vi "ViewData.vi"() -> ()   [LabVIEW 2024]
uses:
  <vilib>/drjdpowell/SQLite Library/SQL Connection/Open (path).vi
  <vilib>/drjdpowell/SQLite Library/SQL Connection/Open (string).vi
  <vilib>/AdvancedString/Path To Command Line String.vi
  <vilib>/drjdpowell/SQLite Library/SQL Connection/Execute SQL (1D String).vi
  <vilib>/drjdpowell/SQLite Library/SQL Connection/Execute SQL (DBL results).vi
  <vilib>/Utility/file.llb/Write Delimited Spreadsheet (DBL).vi
  <vilib>/drjdpowell/SQLite Library/SQL Connection/Connection.lvclass
  <vilib>/drjdpowell/SQLite Library/SQLite.lvlib
panel:
  out "length":i32
  in  "Export Excel":bool
  in  "Export Image Pressure":bool
  in  "Export Excel Pressure":bool
  in  "Export Image Fan":bool
  in  "Export Excel Fan":bool
  out "Data":dbl[][](array[numeric])
  out "Pressure":cluster{dbl[], "Data Table":dbl[]}[](graph)
  out "Fan":cluster{dbl[], "Result Set":dbl[]}[](graph)
  in  "Time":i32(listbox)
  in  "Date":string(combo)
  in  "stop":bool
  out "Time2DArray":string[][](array[string])
  out "DateArray":string[](array[string])
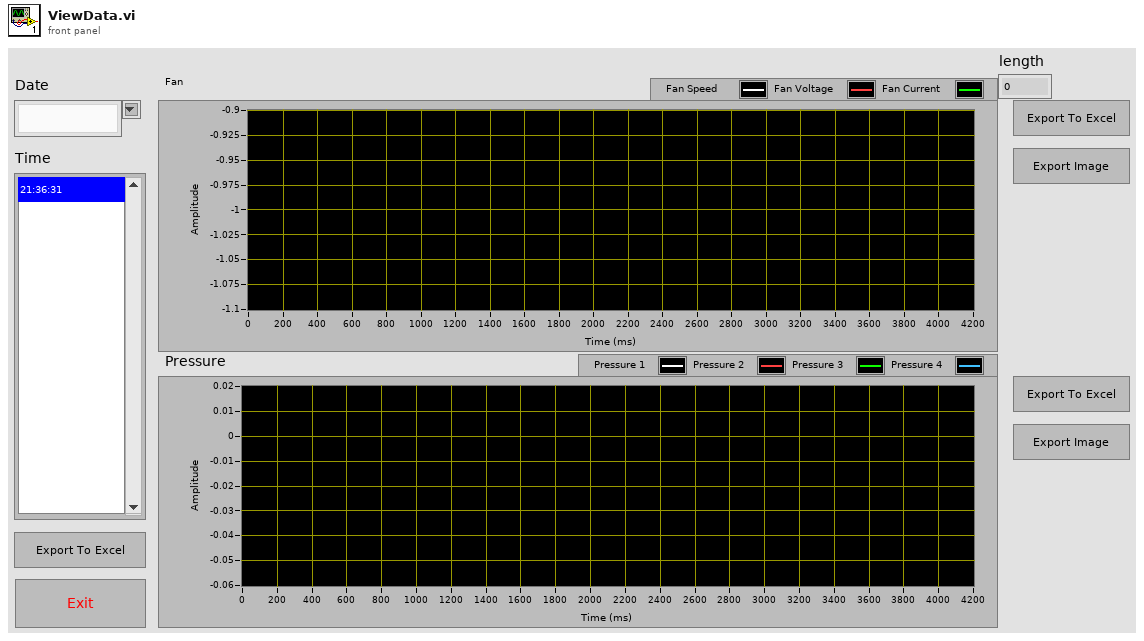
[diagram p1: front panel]
types:
  T1 = enum16{"New or existing", "Existing", "Read only"}
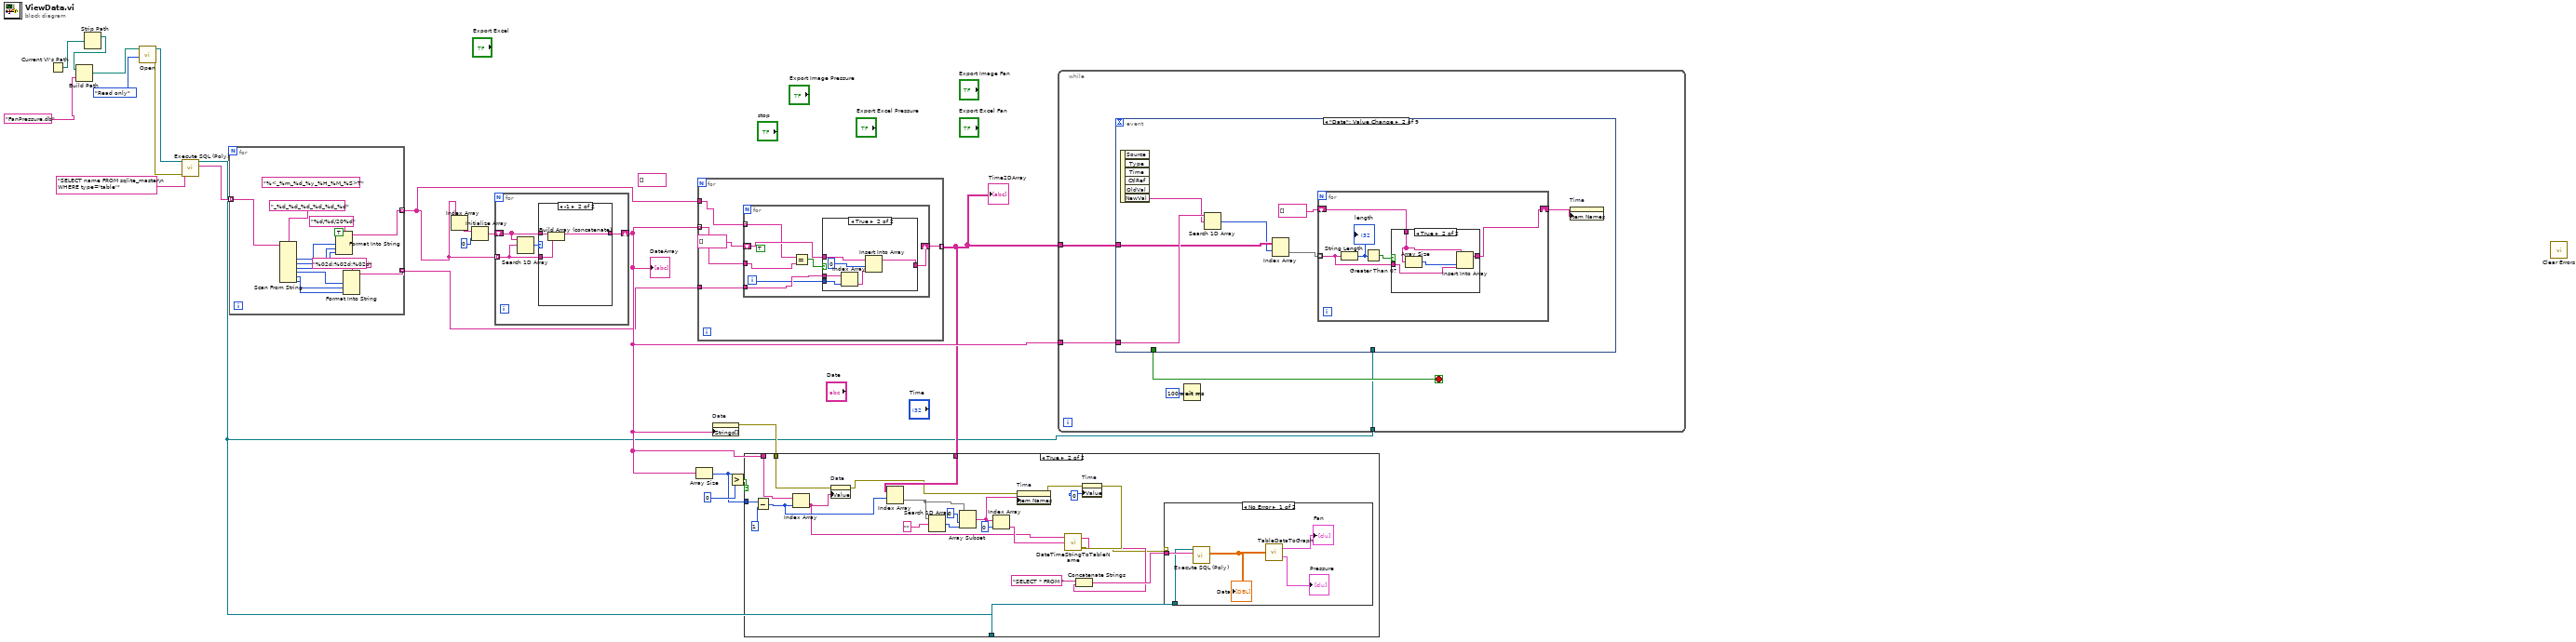
[diagram p0: block diagram]
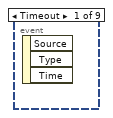
[diagram p4: hidden frame]
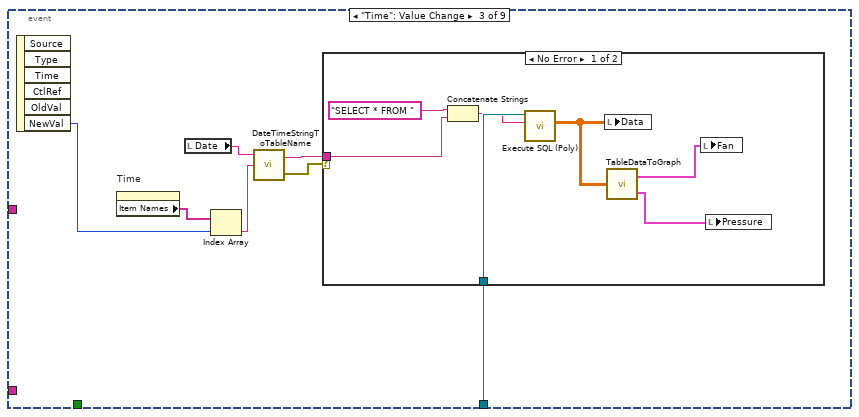
[diagram p6: hidden frame]
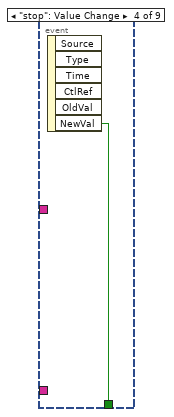
[diagram p8: hidden frame]
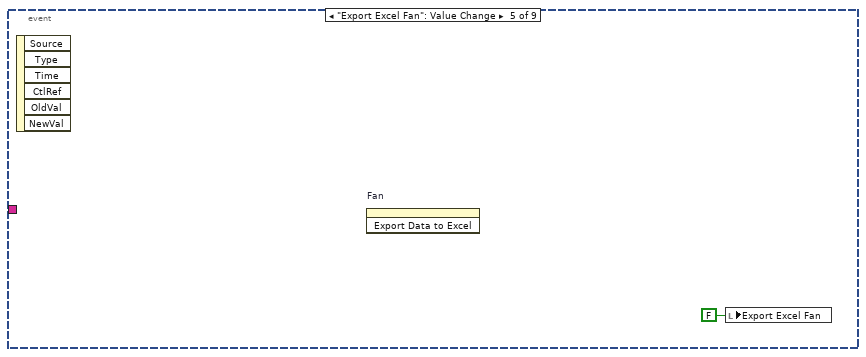
[diagram p9: hidden frame]
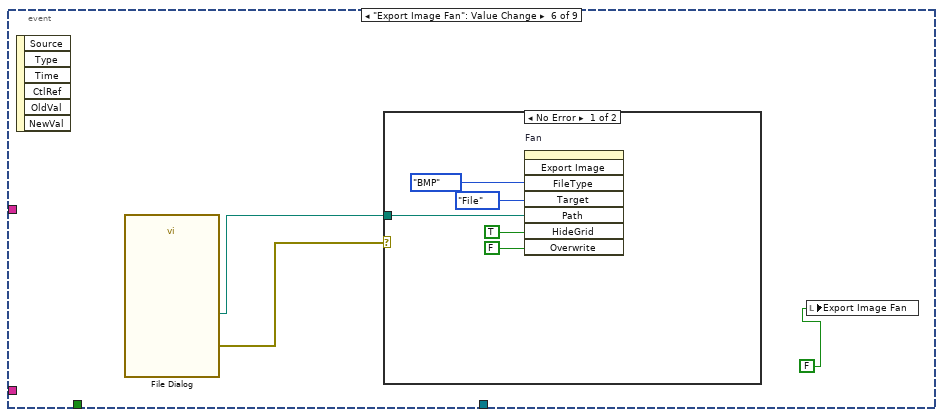
[diagram p10: hidden frame]
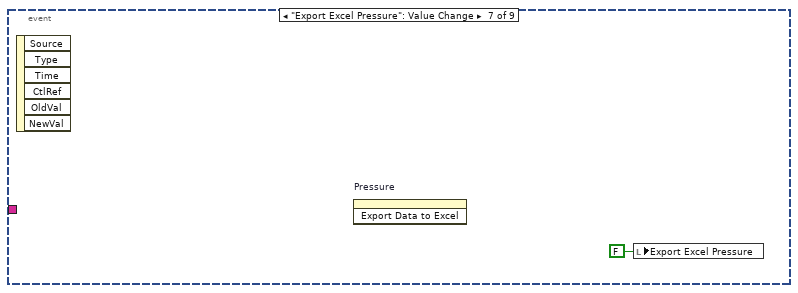
[diagram p12: hidden frame]
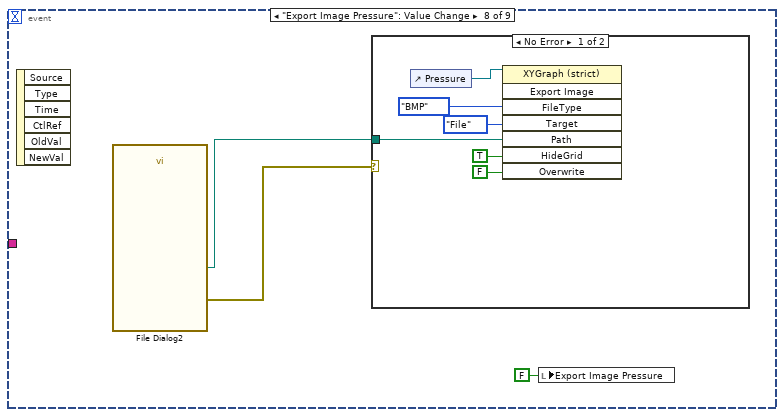
[diagram p13: hidden frame]
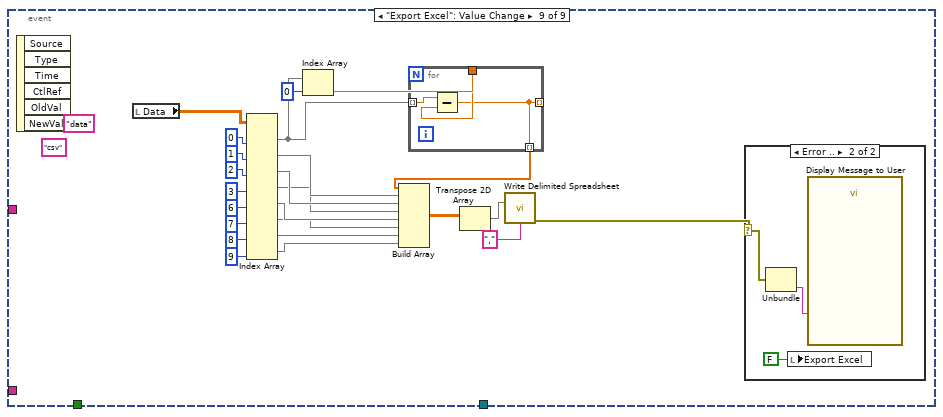
[diagram p15: hidden frame]
diagram:
  (unwired) string[] [] ("Child Text")
  n1 = Current VI's Path() -> (path=w19:path)
  n2 = Strip Path(path=w19) -> (stripped path=w17:path)  [unwired: 1 out]
  n3 = Build Path(base path=w17, name or relative path="FanPressure.db" ("db file")) -> (appended path=w16:path)
  n4 = call-poly <vilib>:"Open.vi"("File Option"=T1."Read only", "db file"=w16) -> ("error out"=w14:errorcluster, "SQLite Connection"=w15:refnum<class "Connection.lvclass">)  [unwired: 8 in]
  n5 = call-poly <vilib>:"Execute SQL (Poly).vi"("error in (no error)"=w14, "SQL"="SELECT name FROM sqlite_master\n    WHERE type='table'", "SQLite Connection in"=w15) -> ("Result Set"=w10:string[], "SQLite Connection"=w1:refnum<class "Connection.lvclass">)  [unwired: 5 in, 2 out]
  n6 = for {
    tunnel: w10 -> [w33] mode=indexing
    tunnel: [w27] -> w3 mode=indexing
    tunnel: [w22] -> w2 mode=indexing
    (unwired) TRUE ("want seconds? (F)")
    (unwired) "%<_%m_%d_%y_%H_%M_%S>T" ("format string")
    n7 = Scan From String(format string="_%d_%d_%d_%d_%d_%d", input string=w33) -> (output 1=w30:i32, output 2=w29:i32, output 3=w28:i32, output 4=w26:i32, output 5=w25:i32, output 6=w24:i32)  [unwired: 8 in, 3 out]
    n8 = Format Into String(format string="%d/%d/20%d", w30, w29, w28) -> (resulting string=w27:string)  [unwired: 2 in, 1 out]
    n9 = Format Into String(format string="%02d:%02d:%02d", w26, w25, w24) -> (resulting string=w22:string)  [unwired: 2 in, 1 out]
  }
  n10 = Index Array(array=w3) -> (element=w11:string)  [unwired: 1 in]
  n11 = Initialize Array(w11, 0 ("Dimension Size")) -> (w12:string[])
  n12 = for {
    tunnel: w3 -> [w36] mode=indexing
    shift-right: [w34] -> w6
    shift-left: w12 -> [w35]
    n13 = Search 1D Array(1D array=w35, element=w36) -> (index of element=w37:i32)  [unwired: 1 in]
    n14 = case shown="-1" w37 {
      tunnel: w36 -> [_ w41]
      tunnel: [w38 w39] -> w34
      tunnel: w35 -> [w38 w40]
      frame Default {
      }
      frame -1 {
        n15 = Build Array (concatenate)(w40, w41) -> (w39:string[])
      }
    }
  }
  "DateArray" <- w6
  n16 = Array Size(array=w6) -> (size(s)=w5:i32)
  n17 = for {
    tunnel: w6 -> [w46] mode=indexing
    tunnel: [w44] -> w4 mode=indexing
    tunnel: w3 -> [w43]
    tunnel: w2 -> [w42]
    n18 = for {
      tunnel: w46 -> [w53]
      shift-right: [w51] -> w44
      shift-left: string[] [] ("Child Text") -> [w52]
      tunnel: w43 -> [w49] mode=indexing
      tunnel: w42 -> [w48]
      i -> [w47]
      (unwired) TRUE ("want seconds? (F)")
      n19 = Equal?(x=w49, y=w53) -> (x = y?=w50:bool)
      n20 = case shown="True" w50 {
        tunnel: w52 -> [w54 w59]
        tunnel: [w54 w58] -> w51
        tunnel: w48 -> [_ w56]
        tunnel: w47 -> [_ w57]
        frame False {
        }
        frame True {
          n21 = Index Array(array=w56, index=w57) -> (element=w55:string)
          n22 = Insert Into Array(array=w59, index=0, new element=w55) -> (w58:string[])
        }
      }
    }
  }
  "Time2DArray" <- w4
  n23 = property on="Date" class="CmbBox"("Strings[]"=w6) -> (error out=w7:errorcluster)  [unwired: 2 in, 1 out]
  n24 = Greater?(x=w5, y=0) -> (0:w8:bool)
  n25 = case shown="True" w8 {
    tunnel: w7 -> [_ w82]
    tunnel: w6 -> [_ w79]
    tunnel: w5 -> [_ w81]
    tunnel: w4 -> [_ w78]
    tunnel: w1 -> [_ w71]
    frame False {
    }
    frame True {
      n26 = Subtract(x=w81, y=1) -> (x-y=w77:i32)
      n27 = Index Array(array=w79, index=w77) -> (element=w69:string)
      n28 = property on="Date" class="CmbBox"(error in=w82, "Value"=w69) -> (error out=w76:errorcluster)  [unwired: 1 in, 1 out]
      n29 = Index Array(array=w78, index (row)=w77) -> (element=w64:string[])  [unwired: 1 in]
      n30 = Search 1D Array(1D array=w64, element="") -> (index of element=w62:i32)  [unwired: 1 in]
      n31 = Array Subset(array=w64, index=0, length=w62) -> (w61:string[])
      n32 = Index Array(array=w61, index=0) -> (element=w70:string)
      n33 = property on="Time" class="LstBox (strict)"(error in=w76, "Item Names"=w61) -> (error out=w68:errorcluster)  [unwired: 1 in, 1 out]
      n34 = call "DateTimeStringToTableName.vi"("error in"=w68, "Time String"=w70, "Date String"=w69) -> ("error out"=w66:errorcluster, "Table Name"=w67:string)
      n35 = Concatenate Strings("SELECT * FROM " ("SQL"), w67) -> (w72:string)
      n36 = property on="Time" class="LstBox (strict)"(error in=w68, "Value"=0 ("Time")) -> ()  [unwired: 1 in, 2 out]
      n37 = case shown="No Error" w66 {
        tunnel: w72 -> [w87 _]
        tunnel: w71 -> [w83 _]
        frame No Error {
          n38 = call-poly <vilib>:"Execute SQL (Poly).vi"("SQL"=w87, "SQLite Connection in"=w83) -> ("Result Set"=w84:dbl[][])  [unwired: 6 in, 3 out]
          "Data" <- w84
          n39 = call "TableDataToGraph.vi"("Data Table"=w84) -> ("Speed Graph"=→"Fan":cluster{dbl[], "Data Table":dbl[]}[], "Pressure Graph"=→"Pressure":cluster{dbl[], "Data Table":dbl[]}[])
        }
        frame Error {
        }
      }
    }
  }
  n40 = while {
    tunnel: w6 -> [w91]
    tunnel: w4 -> [w90]
    tunnel: w1 -> [w88]
    stop <- w89 stop-if-true
    n41 = event shown="[1] \"Date\": Value Change" {
      selector: _ -> [_ _ _ _ _ _ _ _ _]
      dyn-events: _ -> [_ _ _ _ _ _ _ _ _]
      timeout: _ -> [_ _ _ _ _ _ _ _ _]
      tunnel: w91 -> [_ w99 _ _ _ _ _ _ _]
      tunnel: w90 -> [_ w97 _ _ _ _ _ _ _]
      tunnel: [_ _ _ w124 _ _ _ _ _] -> w89
      tunnel: w88 -> [_ _ w114 _ _ _ _ _ _]
      event Timeout {
        n42 = event-data() -> ()  [unwired: 1 in, 3 out]
      }
      event "Date": Value Change {
        n43 = event-data() -> ("NewVal"=w98:string)  [unwired: 1 in, 5 out]
        n44 = Search 1D Array(1D array=w99, element=w98) -> (index of element=w96:i32)  [unwired: 1 in]
        n45 = Index Array(array=w97, index (row)=w96) -> (element=w95:string[])  [unwired: 1 in]
        n46 = for {
          tunnel: w95 -> [w101] mode=indexing
          shift-right: [w100] -> w93
          shift-left: string[] [] ("Item Names") -> [w102]
          n47 = String Length(string=w101) -> (length=w104:i32)
          "length" <- w104
          n48 = Greater Than 0?(x=w104) -> (x > 0?=w103:bool)
          n49 = case shown="True" w103 {
            tunnel: w102 -> [w105 w108]
            tunnel: w101 -> [_ w109]
            tunnel: [w105 w107] -> w100
            frame False {
            }
            frame True {
              n50 = Array Size(array=w108) -> (size(s)=w106:i32)
              n51 = Insert Into Array(array=w108, index=w106, new element=w109) -> (w107:string[])
            }
          }
        }
        n52 = property on="Time" class="LstBox (strict)"("Item Names"=w93) -> ()  [unwired: 2 in, 2 out]
      }
      event "Time": Value Change {
        n53 = event-data() -> ("NewVal"=w115:i32)  [unwired: 1 in, 5 out]
        n54 = property on="Time" class="LstBox (strict)"() -> ("Item Names"=w116:string[])  [unwired: 2 in, 2 out]
        n55 = local read "Date"() -> (w113:string)
        n56 = Index Array(array=w116, index=w115) -> (element=w112:string)
        n57 = call "DateTimeStringToTableName.vi"("Time String"=w112, "Date String"=w113) -> ("error out"=w110:errorcluster, "Table Name"=w111:string)  [unwired: 1 in]
        n58 = case shown="No Error" w110 {
          tunnel: w114 -> [w122 _]
          tunnel: w111 -> [w117 _]
          frame No Error {
            n59 = Concatenate Strings("SELECT * FROM " ("SQL"), w117) -> (w121:string)
            n60 = call-poly <vilib>:"Execute SQL (Poly).vi"("SQL"=w121, "SQLite Connection in"=w122) -> ("Result Set"=w120:dbl[][])  [unwired: 6 in, 3 out]
            n61 = local write "Data"(w120) -> ()
            n62 = call "TableDataToGraph.vi"("Data Table"=w120) -> ("Speed Graph"=w119:cluster{dbl[], "Data Table":dbl[]}[], "Pressure Graph"=w118:cluster{dbl[], "Data Table":dbl[]}[])
            n63 = local write "Fan"(w119) -> ()
            n64 = local write "Pressure"(w118) -> ()
          }
          frame Error {
          }
        }
      }
      event "stop": Value Change {
        n65 = event-data() -> ("NewVal"=w124:bool)  [unwired: 1 in, 5 out]
      }
      event "Export Excel Fan": Value Change {
        n66 = event-data() -> ()  [unwired: 1 in, 6 out]
        n67 = invoke on="Fan" class="XYGraph (strict)" method="Export Data to Excel"() -> ()  [unwired: 3 in, 3 out]
        n68 = local write "Export Excel Fan"(FALSE ("Export Excel Fan")) -> ()
      }
      event "Export Image Fan": Value Change {
        n69 = event-data() -> ()  [unwired: 1 in, 6 out]
        n70 = call "File Dialog"() -> ("selected path"=w128:path, "error out"=w127:errorcluster)  [unwired: 12 in, 2 out]
        n71 = case shown="No Error" w127 {
          tunnel: w128 -> [w129 _]
          frame No Error {
            n72 = invoke on="Fan" class="XYGraph (strict)" method="Export Image"("FileType"=enum32{"BMP", "EPS", "EMF", "PICT"}."BMP" ("File Type"), "Target"=enum32{"File", "Clipboard"}."File", "Path"=w129, "HideGrid"=TRUE ("Hide Grid"), "Overwrite"=FALSE ("Always Overwrite")) -> ()  [unwired: 3 in, 8 out]
          }
          frame Error {
          }
        }
        n73 = local write "Export Image Fan"(FALSE ("Always Overwrite")) -> ()
      }
      event "Export Excel Pressure": Value Change {
        n74 = event-data() -> ()  [unwired: 1 in, 6 out]
        n75 = invoke on="Pressure" class="XYGraph (strict)" method="Export Data to Excel"() -> ()  [unwired: 3 in, 3 out]
        n76 = local write "Export Excel Pressure"(FALSE ("Export Excel Pressure")) -> ()
      }
      event "Export Image Pressure": Value Change {
        n77 = event-data() -> ()  [unwired: 1 in, 6 out]
        n78 = call "File Dialog2"() -> ("selected path"=w137:path, "error out"=w136:errorcluster)  [unwired: 12 in, 2 out]
        n79 = case shown="No Error" w136 {
          tunnel: w137 -> [w139 _]
          frame No Error {
            n80 = control-ref of="Pressure"() -> (w138:refnum<vi>)
            n81 = invoke on="Invoke Node" class="XYGraph (strict)" method="Export Image"(reference=w138, "FileType"=enum32{"BMP", "EPS", "EMF", "PICT"}."BMP" ("File Type"), "Target"=enum32{"File", "Clipboard"}."File", "Path"=w139, "HideGrid"=TRUE ("Hide Grid"), "Overwrite"=FALSE ("Always Overwrite")) -> ()  [unwired: 2 in, 8 out]
          }
          frame Error {
          }
        }
        n82 = local write "Export Image Pressure"(FALSE ("Export Image Pressure")) -> ()
      }
      event "Export Excel": Value Change {
        (unwired) "csv" ("pattern (all files)")
        (unwired) "data" ("default name")
        n83 = event-data() -> ()  [unwired: 1 in, 6 out]
        n84 = local read "Data"() -> (w167:dbl[][])
        n85 = Index Array(array=w167, index (col) #1=0 ("disabled index (col)"), index (col) #2=1 ("index (col)"), index (col) #3=2 ("index (col)"), index (col) #4=3 ("index (col)"), index (col) #5=6 ("index (col)"), index (col) #6=7 ("index (col)"), index (col) #7=8 ("index (col)"), index (col) #8=9 ("index (col)")) -> (element #1=w149:dbl[], element #2=w158:dbl[], element #3=w157:dbl[], element #4=w156:dbl[], element #5=w155:dbl[], element #6=w154:dbl[], element #7=w153:dbl[], element #8=w152:dbl[])  [unwired: 8 in]
        n86 = Index Array(array=w149, index=0) -> (element=w147:dbl)
        n87 = for {
          tunnel: w149 -> [w171] mode=indexing
          tunnel: w147 -> [w170]
          tunnel: [w169] -> _ mode=indexing
          tunnel: [w169] -> w146 mode=indexing
          n88 = Subtract(x=w171, y=w170) -> (x-y=w169:dbl)
        }
        n89 = Build Array(w146, w158, w157, w156, w155, w154, w153, w152) -> (w145:dbl[][])
        n90 = Transpose 2D Array(2D array=w145) -> (transposed array=w144:dbl[][])
        n91 = call-poly <vilib>:"Write Delimited Spreadsheet.vi"("2D data"=w144, "delimiter (\\t)"="," ("delimiter (\\t)")) -> ("error out"=w150:errorcluster)  [unwired: 12 in, 1 out]
        n92 = case shown="Error .." w150 {
          selector: w150 -> [_ w173]
          frame No Error {
          }
          frame Error {
            n93 = Unbundle(w173) -> ("source"=w172:string)  [unwired: 2 out]
            n94 = call "Display Message to User"("Message"=w172) -> ()  [unwired: 9 in, 2 out]
          }
        }
        n95 = local write "Export Excel"(FALSE ("Export Excel")) -> ()
      }
    }
    n96 = Wait (ms)(milliseconds to wait=u32 100) -> ()  [unwired: 1 out]
  }
  n97 = call <vilib>:"Clear Errors.vi"() -> ()  [unwired: 6 in, 2 out]
